vi "Memory.Pointer.Internal.New.vi"(8 "error in (no error)":errorcluster, 11 "size":u64 format="%08x bytes") -> (0 "error out":errorcluster, 3 "pointer":refnum<class "Memory.Pointer.Internal.lvclass">)   [LabVIEW 2016, in "Memory Manager.lvlib" / "Memory.Pointer.Internal.lvclass"]
doc: "Allocates a new pointer that points to a block of memory that is <b>size</b> bytes in length."
uses:
  Memory.Pointer.Internal.lvclass
  C:/Git/SourceTree/LabVIEW-Memory-Manager/Source/Classes/Pointer/Memory.Pointer.lvclass
  Pointer/Memory.Pointer.lvclass/Memory.Pointer.ctl
  Pointer/Memory.Pointer.lvclass
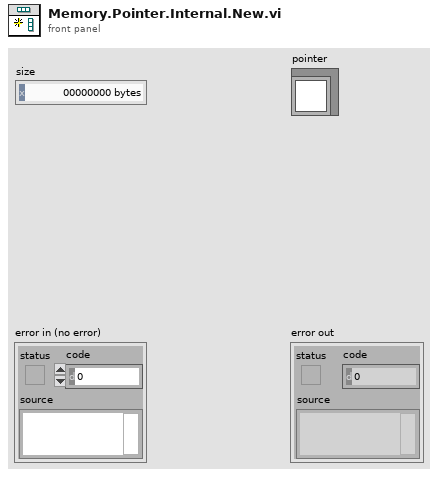
[diagram p1: front panel]
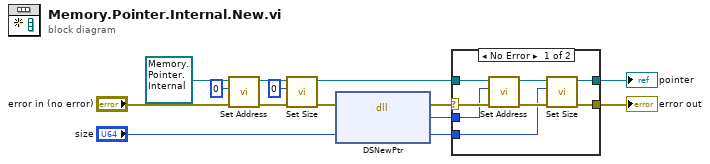
[diagram p0: block diagram]
diagram:
  n1 = call "Set Address.vi"("error in (no error)"="error in (no error)", "address"=u64 0, "Pointer in"=refnum<class "Memory.Pointer.Internal.lvclass"> refnum ("Pointer")) -> ("error out"=w2:errorcluster, "Pointer out"=w9:refnum<class "Memory.Pointer.Internal.lvclass">)  [unwired: 7 in]
  n2 = call "Set Size.vi"("error in (no error)"=w2, "size"=u64 0, "Pointer in"=w9) -> ("error out"=w1:errorcluster, "Pointer out"=w8:refnum<class "Memory.Pointer.Internal.lvclass">)  [unwired: 7 in]
  n3 = dll-call lib="LabVIEW" fn="DSNewPtr"(error in=w1, "size"="size") -> (error out=w5:errorcluster, "pointer"=w7:u64, "size"=w6:u64)  [unwired: 2 in, 1 out]
  n4 = case shown="No Error" w5 {
    selector: w5 -> [w21 w23]
    tunnel: w8 -> [w22 w24]
    tunnel: w7 -> [w20 _]
    tunnel: [w17 w24] -> w14
    tunnel: w6 -> [w15 _]
    tunnel: [w16 w23] -> w4
    frame No Error {
      n5 = call "Set Address.vi"("error in (no error)"=w21, "address"=w20, "Pointer in"=w22) -> ("error out"=w18:errorcluster, "Pointer out"=w19:refnum<class "Memory.Pointer.Internal.lvclass">)  [unwired: 7 in]
      n6 = call "Set Size.vi"("error in (no error)"=w18, "size"=w15, "Pointer in"=w19) -> ("error out"=w16:errorcluster, "Pointer out"=w17:refnum<class "Memory.Pointer.Internal.lvclass">)  [unwired: 7 in]
    }
    frame Error {
    }
  }
  "error out" <- w4
  "pointer" <- w14
